vi "writeInCSV.vi"() -> ()   [LabVIEW 2019]
uses:
  c0fc650a-b9ce-4c6e-94f0-9ae501e176ac.vi
  <vilib>/Utility/file.llb/Write Delimited Spreadsheet (string).vi
panel:
  in  "Container":cluster{"Temp Data":dbl, "Message":string}[](array[cluster])
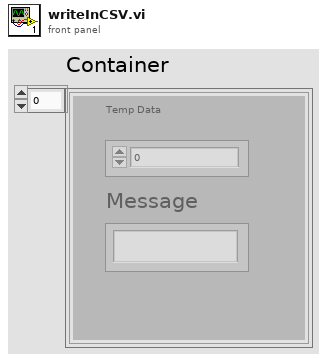
[diagram p1: front panel]
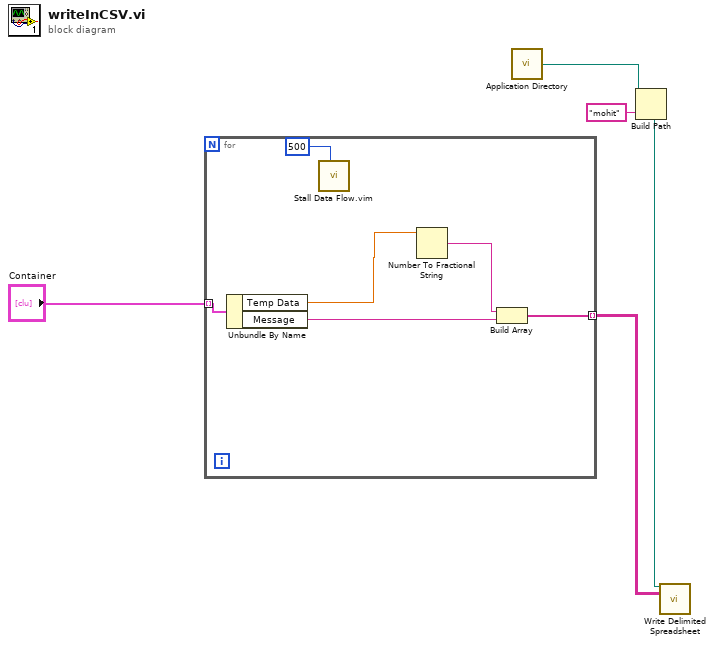
[diagram p0: block diagram]
diagram:
  n1 = for {
    tunnel: "Container" -> [w11] mode=indexing
    tunnel: [w7] -> w4 mode=indexing
    n2 = Unbundle By Name(w11) -> ("Temp Data"=w10:dbl, "Message"=w8:string)
    n3 = call "Stall Data Flow.vim"("milliseconds to wait"=u32 500) -> ()  [unwired: 1 in, 2 out]
    n4 = Number To Fractional String(number=w10) -> (F-format string=w9:string)  [unwired: 3 in]
    n5 = Build Array(w9, w8) -> (w7:string[])
  }
  n6 = call <vilib>:"Application Directory.vi"() -> ("Application Directory"=w3:path)
  n7 = Build Path(base path=w3, name or relative path="mohit") -> (appended path=w2:path)
  n8 = call-poly <vilib>:"Write Delimited Spreadsheet.vi"("file path (dialog if empty)"=w2, "2D data"=w4) -> ()  [unwired: 12 in, 2 out]
